vi "mbed-write Hello World.vi"() -> ()   [LabVIEW 2016]
panel:
  in  "Serial Port":refnum<visa-resource-name>
  in  "LED2":dbl(slide) scale=0.0..1.0
  out "The String output to mbed":string
  in  "stop":bool
  in  "LED1":dbl(slide) scale=0.0..1.0
  # "mbed-write Hello World!"
  # "http://mbed.org"
  # "Note: The mbed-write VI adds the termination character"
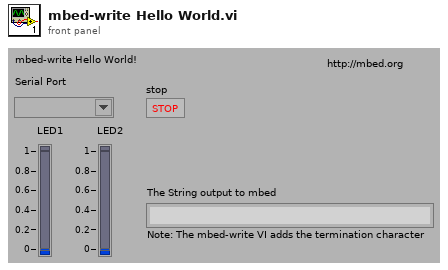
[diagram p1: front panel]
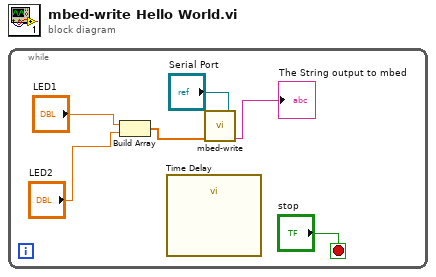
[diagram p0: block diagram]
diagram:
  n1 = while {
    stop <- "stop" stop-if-true
    n2 = Build Array("LED1", "LED2") -> (w3:dbl[])
    n3 = call "Time Delay"() -> ()  [unwired: 11 in, 1 out]
    n4 = call "mbed-write.vi"("Serial Port"="Serial Port", "Array of Numbers"=w3) -> ("Write Output"=→"The String output to mbed":string)  [unwired: 5 in]
  }
